vi "AutoRoutinePreProcessor.vi"(1 "MotionPlanningNotifiers":T1, 2 "RawSteps":T11[](array[typedef])) -> (0 "PreProcessedSteps":T2[](array[typedef]) {"ArmPath"."ExtendTrajectory"."Time (ms)" items=["TrajectoryDuration_0ms"=0, "TrajectoryDuration_5ms"=5, "TrajectoryDuration_10ms"=10, "TrajectoryDuration_20ms"=20, "TrajectoryDuration_30ms"=30, "TrajectoryDuration_40ms"=40, "TrajectoryDuration_50ms"=50, "TrajectoryDuration_100ms"=100]; "ArmPath"."RotateTrajectory"."Time (ms)" items=["TrajectoryDuration_0ms"=0, "TrajectoryDuration_5ms"=5, "TrajectoryDuration_10ms"=10, "TrajectoryDuration_20ms"=20, "TrajectoryDuration_30ms"=30, "TrajectoryDuration_40ms"=40, "TrajectoryDuration_50ms"=50, "TrajectoryDuration_100ms"=100]})   [LabVIEW 2017]
uses:
  TypeDef/AutoStep.ctl
  TypeDef/AutoWaypointType.ctl
  Pathfinder/Pathfinder-LabVIEW/Pathfinder-Lib/VIs/Waypoint.ctl
  Implements/Arm/TypeDefs/ArmTargetPosition.ctl
  Implements/TypeDefs/IntakeState.ctl
  TypeDef/AutoPreProcessedStep.ctl
  PathPlannerSupport/TypeDefs/DrivePlanResponse.ctl
  Pathfinder/Pathfinder-LabVIEW/Pathfinder-Lib/VIs/Segment.ctl
  Implements/Arm/TypeDefs/ArmPlanResponse.ctl
  General/MotionProfiling/TypeDefs/TrajectoryPoint.ctl
  <vilib>/Rock Robotics/WPI/ThirdParty/Phoenix-LabVIEW/Motor Controller/Controls/CTRE_Phoenix_MotorControl_TrajectoryPointTimeDur.ctl
  TypeDefs/RobotComponents/MotionPlanningNotifiers.ctl
  PathPlannerSupport/TypeDefs/DrivePlanRequest.ctl
  Implements/Arm/TypeDefs/ArmPlanRequest.ctl
  Pathfinder/Pathfinder-LabVIEW/Pathfinder-Lib/Pathfinder.lvlib
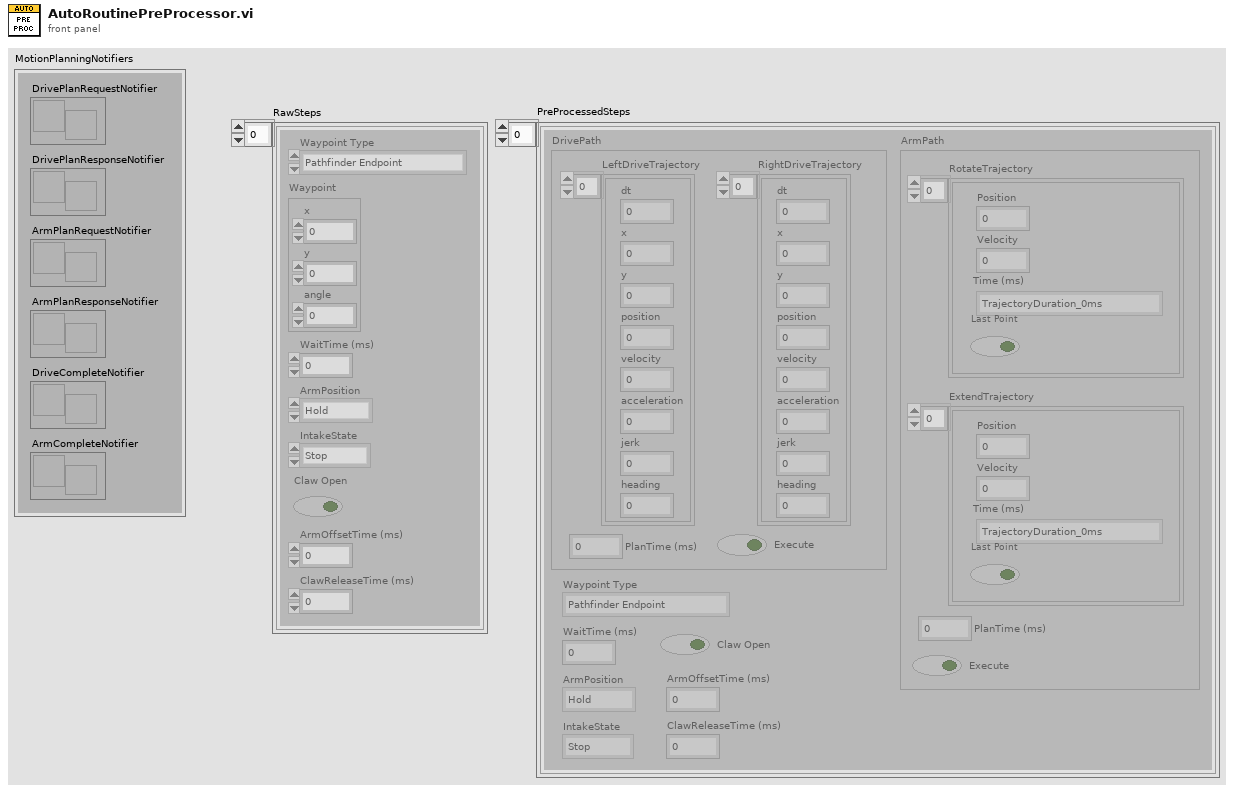
[diagram p1: front panel]
types:
  T1 = typedef "MotionPlanningNotifiers.ctl" = cluster{"DrivePlanRequestNotifier":refnum<notifier>, "DrivePlanResponseNotifier":refnum<notifier>, "ArmPlanRequestNotifier":refnum<notifier>, "ArmPlanResponseNotifier":refnum<notifier>, "DriveCompleteNotifier":refnum<notifier>, "ArmCompleteNotifier":refnum<notifier>}
  T2 = typedef "AutoPreProcessedStep.ctl" = cluster{"DrivePath":T3, "ArmPath":T5, "Waypoint Type":T8, "WaitTime (ms)":u16, "ArmPosition":T9, "IntakeState":T10, "Claw Open":bool, "ArmOffsetTime (ms)":u16, "ClawReleaseTime (ms)":i32}
  T3 = typedef "DrivePlanResponse.ctl" = cluster{"LeftDriveTrajectory":T4[], "RightDriveTrajectory":T4[], "PlanTime (ms)":u32, "Execute":bool}
  T4 = typedef "Pathfinder.lvlib/Segment.ctl" = cluster{"dt":dbl, "x":dbl, "y":dbl, "position":dbl, "velocity":dbl, "acceleration":dbl, "jerk":dbl, "heading":dbl}
  T5 = typedef "ArmPlanResponse.ctl" = cluster{"RotateTrajectory":T6[], "ExtendTrajectory":T6[], "PlanTime (ms)":u32, "Execute":bool}
  T6 = typedef "TrajectoryPoint.ctl" = cluster{"Position ":dbl, "Velocity ":dbl, "Time (ms)":T7, "Last Point":bool}
  T7 = typedef "CTRE_Phoenix_MotorControl_TrajectoryPointTimeDur.ctl" = i32
  T8 = typedef "AutoWaypointType.ctl" = enum16{"Pathfinder Endpoint", "Pathfinder Waypoint", "Zero-Radius Turn Endpoint", "Stationary", "Vision Assist Endpoint", "Stop"}
  T9 = typedef "ArmTargetPosition.ctl" = enum16{"Hold", "Switch", "Scale Low", "Scale High", "Climb", "Back Place"}
  T10 = typedef "IntakeState.ctl" = enum16{"Stop", "Forward", "Reverse", "Forward Open"}
  T11 = typedef "AutoStep.ctl" = cluster{"Waypoint Type":T8, "Waypoint":T12, "WaitTime (ms)":u16, "ArmPosition":T9, "IntakeState":T10, "Claw Open":bool, "ArmOffsetTime (ms)":u16, "ClawReleaseTime (ms)":i32}
  T12 = typedef "Pathfinder.lvlib/Waypoint.ctl" = cluster{"x":dbl, "y":dbl, "angle":dbl}
  T13 = typedef "ArmPlanRequest.ctl" = cluster{"Destination":T9, "Preview":bool, "Start":T9, "Fixed Start":bool}
  T14 = typedef "DrivePlanRequest.ctl" = cluster{"Plan Type":T8, "Waypoints":T12[], "Preview":bool}
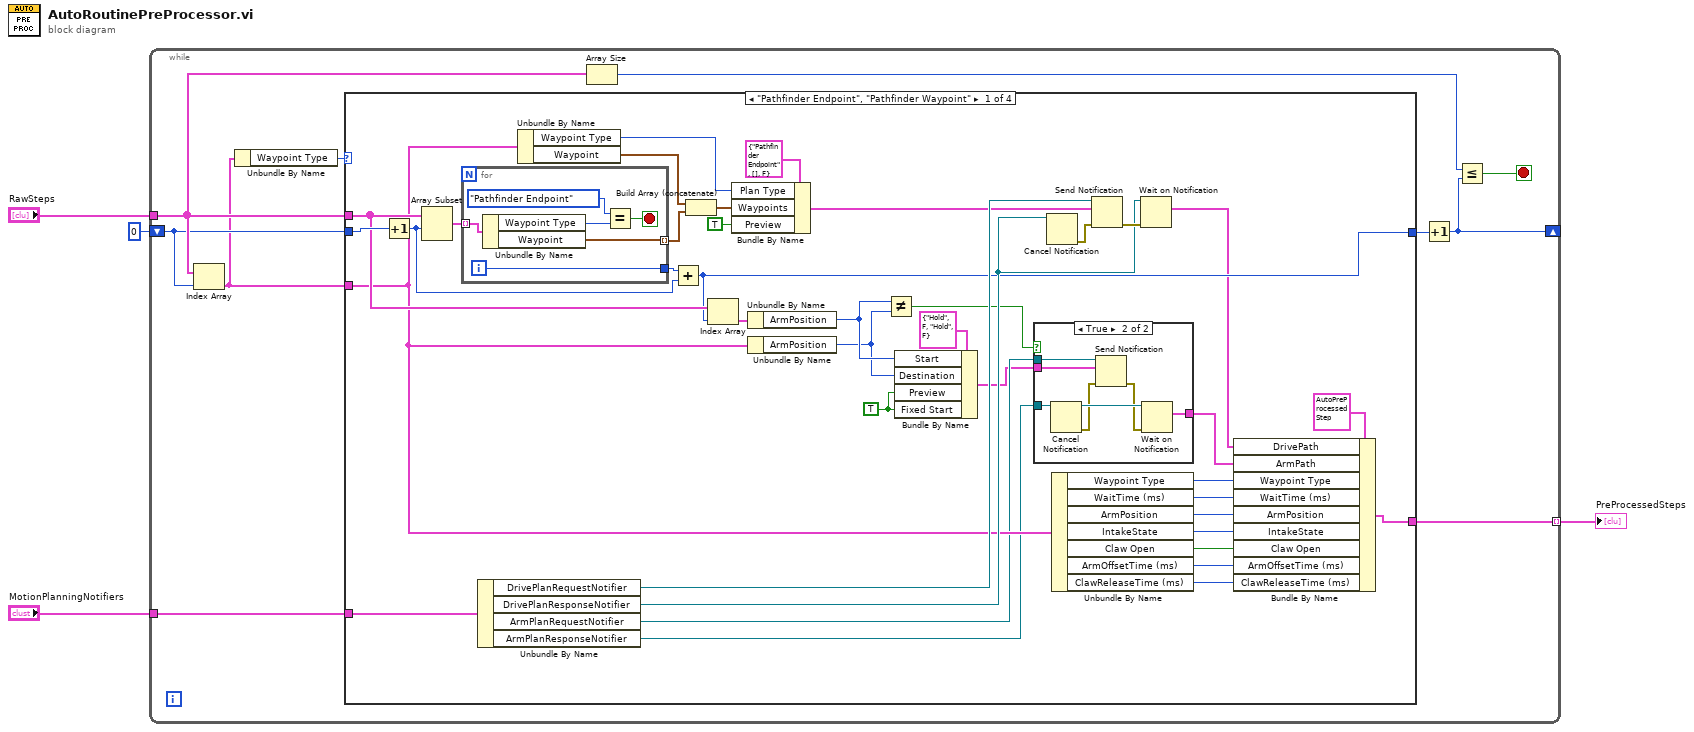
[diagram p0: block diagram]
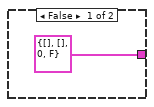
[diagram p2: hidden frame]
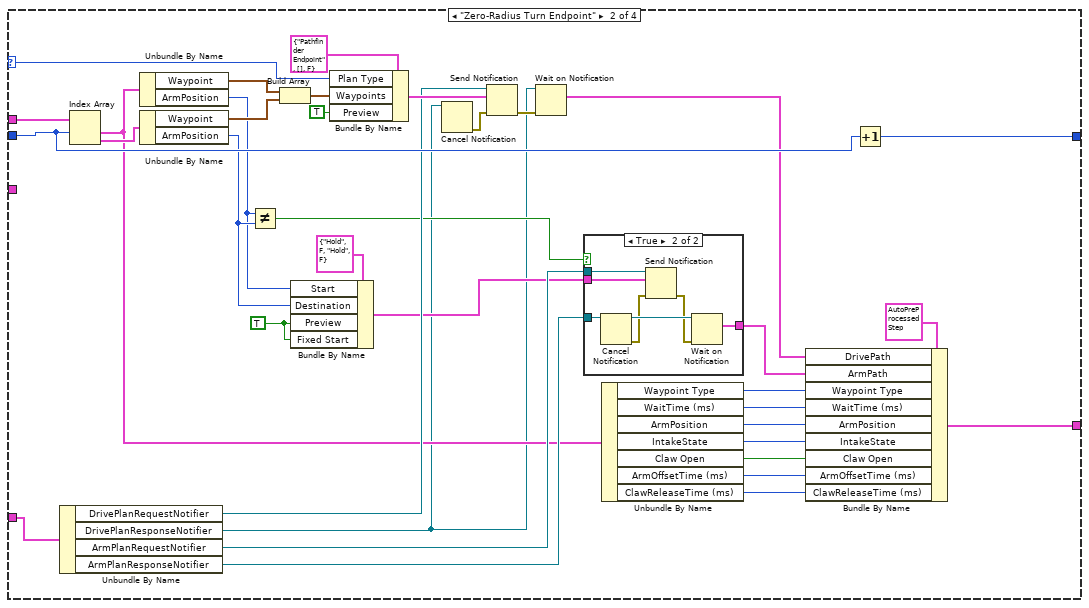
[diagram p3: hidden frame]
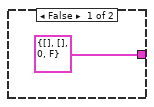
[diagram p4: hidden frame]
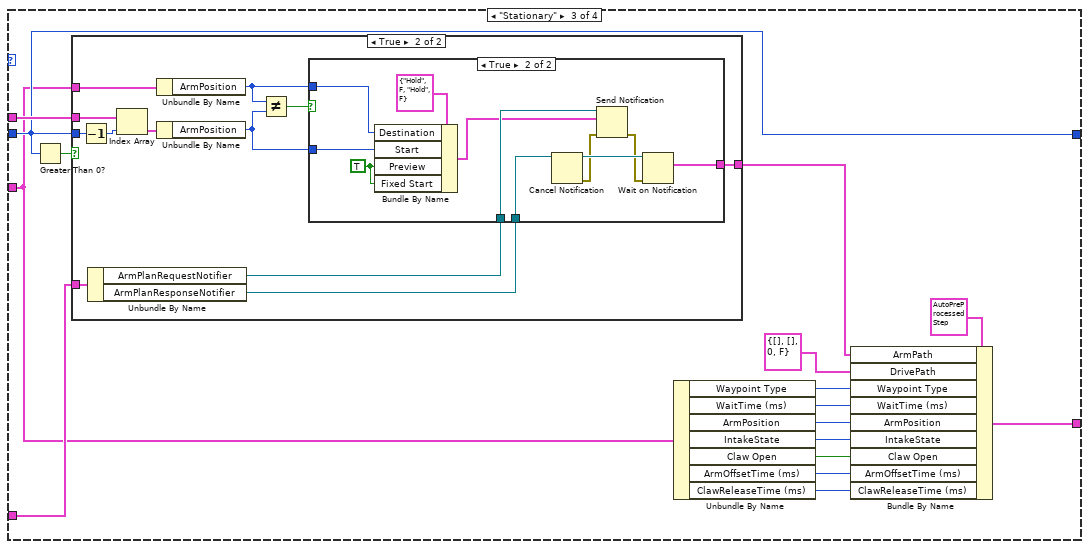
[diagram p5: hidden frame]
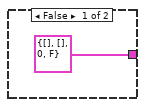
[diagram p6: hidden frame]
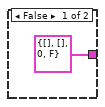
[diagram p7: hidden frame]
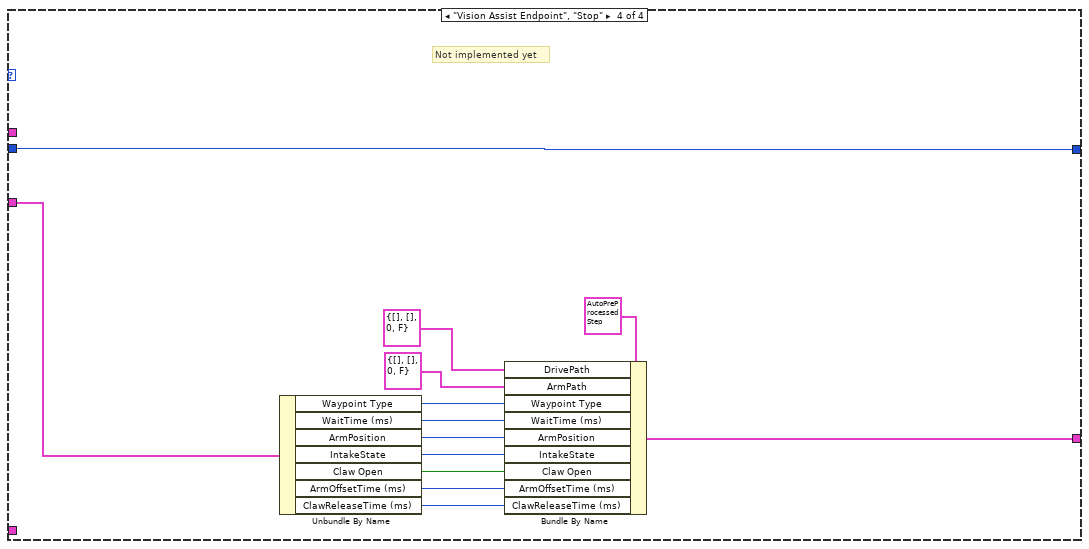
[diagram p8: hidden frame]
diagram:
  n1 = while {
    tunnel: "RawSteps" -> [w9]
    tunnel: "MotionPlanningNotifiers" -> [w14]
    shift-right: [w12] -> _
    shift-left: 0 -> [w8]
    tunnel: [w7] -> w1 mode=indexing
    stop <- w10 stop-if-true
    n2 = Index Array(array=w9, index=w8) -> (element=w6:T11)
    n3 = Unbundle By Name(w6) -> ("Waypoint Type"=w5:T8)
    n4 = case shown="\"Pathfinder Endpoint\", \"Pathfinder Waypoint\"" w5 {
      selector: w5 -> [_ w72 _ _]
      tunnel: w9 -> [w41 w103 w126 _]
      tunnel: w8 -> [w42 w101 w124 w165]
      tunnel: w6 -> [w24 _ w123 w162]
      tunnel: [w18 w102 w124 w165] -> w13
      tunnel: w14 -> [w43 w94 w125 _]
      tunnel: [w19 w71 w121 w163] -> w7
      frame "Pathfinder Endpoint", "Pathfinder Waypoint" {
        w15 = TRUE ("Preview")
        n5 = Increment(x=w42) -> (x+1=w51:i32)
        n6 = Array Subset(array=w41, index=w51) -> (w53:T11[])  [unwired: 1 in]
        n7 = for {
          tunnel: w53 -> [w67] mode=indexing
          tunnel: [w63] -> w52
          tunnel: [w62] -> w47 mode=indexing
          i -> [w63]
          stop <- w64 stop-if-true
          n8 = Unbundle By Name(w67) -> ("Waypoint Type"=w66:T8, "Waypoint"=w62:T12)
          n9 = Equal?(x=AutoWaypointType."Pathfinder Endpoint", y=w66) -> (x = y?=w64:bool)
        }
        n10 = Unbundle By Name(w43) -> ("DrivePlanRequestNotifier"=w36:refnum<notifier>, "DrivePlanResponseNotifier"=w35:refnum<notifier>, "ArmPlanRequestNotifier"=w21:refnum<notifier>, "ArmPlanResponseNotifier"=w22:refnum<notifier>)
        n11 = Unbundle By Name(w24) -> ("Waypoint Type"=w49:T8, "Waypoint"=w48:T12)
        n12 = Add(x=w52, y=w51) -> (x+y=w18:i32)
        n13 = Build Array (concatenate)(w48, w47) -> (w46:T12[])
        n14 = Index Array(array=w41, index=w18) -> (element=w40:T11)
        n15 = Bundle By Name(cluster=T14 {"Plan Type"=enum."Pathfinder Endpoint", "Waypoints"=[], "Preview"=FALSE} ("DrivePlanRequest"), "Plan Type"=w49, "Waypoints"=w46, "Preview"=TRUE) -> (w34:T14)
        n16 = Unbundle By Name(w40) -> ("ArmPosition"=w39:T9)
        n17 = Unbundle By Name(w24) -> ("ArmPosition"=w16:T9)
        n18 = Not Equal?(x=w39, y=w16) -> (x != y?=w23:bool)
        n19 = Bundle By Name(cluster=T13 {"Destination"=enum."Hold", "Preview"=FALSE, "Start"=enum."Hold", "Fixed Start"=FALSE} ("ArmPlanRequest"), "Start"=w39, "Destination"=w16, "Preview"=w15, "Fixed Start"=w15) -> (w20:T13)
        n20 = case shown="True" w23 {
          tunnel: w21 -> [_ w61]
          tunnel: w20 -> [_ w60]
          tunnel: w22 -> [_ w59]
          tunnel: [T5 {"RotateTrajectory"=[], "ExtendTrajectory"=[], "PlanTime (ms)"=0, "Execute"=FALSE} ("ArmPlanResponse") w55] -> w26
          frame False {
          }
          frame True {
            n21 = Cancel Notification(0:w59) -> (8:w58:refnum<notifier>, 11:w57:errorcluster)  [unwired: 1 in, 1 out]
            n22 = Send Notification(notification=w60, notifier=w61, error in (no error)=w57) -> (error out=w56:errorcluster)  [unwired: 1 out]
            n23 = Wait on Notification(notifier=w58, error in (no error)=w56) -> (notification=w55:T5)  [unwired: 2 in, 3 out]
          }
        }
        n24 = Cancel Notification(0:w35) -> (11:w37:errorcluster)  [unwired: 1 in, 2 out]
        n25 = Unbundle By Name(w24) -> ("Waypoint Type"=w25:T8, "WaitTime (ms)"=w27:u16, "ArmPosition"=w28:T9, "IntakeState"=w29:T10, "Claw Open"=w30:bool, "ArmOffsetTime (ms)"=w31:u16, "ClawReleaseTime (ms)"=w32:i32)
        n26 = Send Notification(notification=w34, notifier=w36, error in (no error)=w37) -> (error out=w38:errorcluster)  [unwired: 1 out]
        n27 = Wait on Notification(notifier=w35, error in (no error)=w38) -> (notification=w17:T3)  [unwired: 2 in, 3 out]
        n28 = Bundle By Name(cluster=T2 {"DrivePath"={"LeftDriveTrajectory"=[], "RightDriveTrajectory"=[], "PlanTime (ms)"=0, "Execute"=FALSE}, "ArmPath"={"RotateTrajectory"=[], "ExtendTrajectory"=[], "PlanTime (ms)"=0, "Execute"=FALSE}, "Waypoint Type"=enum."Pathfinder Endpoint", "WaitTime (ms)"=0, "ArmPosition"=enum."Hold", "IntakeState"=enum."Stop", "Claw Open"=FALSE, "ArmOffsetTime (ms)"=0, "ClawReleaseTime (ms)"=0} ("Cluster"), "DrivePath"=w17, "ArmPath"=w26, "Waypoint Type"=w25, "WaitTime (ms)"=w27, "ArmPosition"=w28, "IntakeState"=w29, "Claw Open"=w30, "ArmOffsetTime (ms)"=w31, "ClawReleaseTime (ms)"=w32) -> (w19:T2)
      }
      frame "Zero-Radius Turn Endpoint" {
        w80 = TRUE ("Preview")
        n29 = Unbundle By Name(w94) -> ("DrivePlanRequestNotifier"=w93:refnum<notifier>, "DrivePlanResponseNotifier"=w82:refnum<notifier>, "ArmPlanRequestNotifier"=w91:refnum<notifier>, "ArmPlanResponseNotifier"=w87:refnum<notifier>)
        n30 = Index Array(array=w103, index #1=w101) -> (element #1=w85:T11, element #2=w86:T11)  [unwired: 1 in]
        n31 = Unbundle By Name(w85) -> ("Waypoint"=w99:T12, "ArmPosition"=w81:T9)
        n32 = Unbundle By Name(w86) -> ("Waypoint"=w98:T12, "ArmPosition"=w89:T9)
        n33 = Not Equal?(x=w81, y=w89) -> (x != y?=w88:bool)
        n34 = Build Array(w99, w98) -> (w97:T12[])
        n35 = Bundle By Name(cluster=T13 {"Destination"=enum."Hold", "Preview"=FALSE, "Start"=enum."Hold", "Fixed Start"=FALSE} ("ArmPlanRequest"), "Start"=w81, "Destination"=w89, "Preview"=w80, "Fixed Start"=w80) -> (w90:T13)
        n36 = Bundle By Name(cluster=T14 {"Plan Type"=enum."Pathfinder Endpoint", "Waypoints"=[], "Preview"=FALSE} ("DrivePlanRequest"), "Plan Type"=w72, "Waypoints"=w97, "Preview"=TRUE) -> (w96:T14)
        n37 = Cancel Notification(0:w82) -> (11:w83:errorcluster)  [unwired: 1 in, 2 out]
        n38 = Send Notification(notification=w96, notifier=w93, error in (no error)=w83) -> (error out=w84:errorcluster)  [unwired: 1 out]
        n39 = Wait on Notification(notifier=w82, error in (no error)=w84) -> (notification=w70:T3)  [unwired: 2 in, 3 out]
        n40 = case shown="True" w88 {
          tunnel: w91 -> [_ w111]
          tunnel: w90 -> [_ w110]
          tunnel: w87 -> [_ w109]
          tunnel: [T5 {"RotateTrajectory"=[], "ExtendTrajectory"=[], "PlanTime (ms)"=0, "Execute"=FALSE} ("ArmPlanResponse") w105] -> w69
          frame False {
          }
          frame True {
            n41 = Cancel Notification(0:w109) -> (8:w108:refnum<notifier>, 11:w107:errorcluster)  [unwired: 1 in, 1 out]
            n42 = Send Notification(notification=w110, notifier=w111, error in (no error)=w107) -> (error out=w106:errorcluster)  [unwired: 1 out]
            n43 = Wait on Notification(notifier=w108, error in (no error)=w106) -> (notification=w105:T5)  [unwired: 2 in, 3 out]
          }
        }
        n44 = Unbundle By Name(w85) -> ("Waypoint Type"=w68:T8, "WaitTime (ms)"=w73:u16, "ArmPosition"=w74:T9, "IntakeState"=w75:T10, "Claw Open"=w76:bool, "ArmOffsetTime (ms)"=w77:u16, "ClawReleaseTime (ms)"=w78:i32)
        n45 = Bundle By Name(cluster=T2 {"DrivePath"={"LeftDriveTrajectory"=[], "RightDriveTrajectory"=[], "PlanTime (ms)"=0, "Execute"=FALSE}, "ArmPath"={"RotateTrajectory"=[], "ExtendTrajectory"=[], "PlanTime (ms)"=0, "Execute"=FALSE}, "Waypoint Type"=enum."Pathfinder Endpoint", "WaitTime (ms)"=0, "ArmPosition"=enum."Hold", "IntakeState"=enum."Stop", "Claw Open"=FALSE, "ArmOffsetTime (ms)"=0, "ClawReleaseTime (ms)"=0} ("Cluster"), "DrivePath"=w70, "ArmPath"=w69, "Waypoint Type"=w68, "WaitTime (ms)"=w73, "ArmPosition"=w74, "IntakeState"=w75, "Claw Open"=w76, "ArmOffsetTime (ms)"=w77, "ClawReleaseTime (ms)"=w78) -> (w71:T2)
        n46 = Increment(x=w101) -> (x+1=w102:i32)
      }
      frame "Stationary" {
        n47 = Greater Than 0?(x=w124) -> (x > 0?=w127:bool)
        n48 = case shown="True" w127 {
          tunnel: w126 -> [_ w140]
          tunnel: w124 -> [_ w139]
          tunnel: w123 -> [_ w136]
          tunnel: w125 -> [_ w134]
          tunnel: [T5 {"RotateTrajectory"=[], "ExtendTrajectory"=[], "PlanTime (ms)"=0, "Execute"=FALSE} ("ArmPlanResponse") w129] -> w113
          frame False {
          }
          frame True {
            n49 = Decrement(x=w139) -> (x-1=w138:i32)
            n50 = Unbundle By Name(w134) -> ("ArmPlanRequestNotifier"=w133:refnum<notifier>, "ArmPlanResponseNotifier"=w131:refnum<notifier>)
            n51 = Index Array(array=w140, index=w138) -> (element=w137:T11)
            n52 = Unbundle By Name(w136) -> ("ArmPosition"=w132:T9)
            n53 = Unbundle By Name(w137) -> ("ArmPosition"=w130:T9)
            n54 = Not Equal?(x=w132, y=w130) -> (x != y?=w135:bool)
            n55 = case shown="True" w135 {
              tunnel: w133 -> [_ w148]
              tunnel: w132 -> [_ w145]
              tunnel: w131 -> [_ w147]
              tunnel: w130 -> [_ w144]
              tunnel: [T5 {"RotateTrajectory"=[], "ExtendTrajectory"=[], "PlanTime (ms)"=0, "Execute"=FALSE} ("ArmPlanResponse") w142] -> w129
              frame False {
              }
              frame True {
                w143 = TRUE ("Preview")
                n56 = Bundle By Name(cluster=T13 {"Destination"=enum."Hold", "Preview"=FALSE, "Start"=enum."Hold", "Fixed Start"=FALSE} ("notification"), "Destination"=w145, "Start"=w144, "Preview"=w143, "Fixed Start"=w143) -> (w146:T13)
                n57 = Cancel Notification(0:w147) -> (8:w151:refnum<notifier>, 11:w150:errorcluster)  [unwired: 1 in, 1 out]
                n58 = Send Notification(notification=w146, notifier=w148, error in (no error)=w150) -> (error out=w149:errorcluster)  [unwired: 1 out]
                n59 = Wait on Notification(notifier=w151, error in (no error)=w149) -> (notification=w142:T5)  [unwired: 2 in, 3 out]
              }
            }
          }
        }
        n60 = Unbundle By Name(w123) -> ("Waypoint Type"=w112:T8, "WaitTime (ms)"=w115:u16, "ArmPosition"=w116:T9, "IntakeState"=w117:T10, "Claw Open"=w118:bool, "ArmOffsetTime (ms)"=w119:u16, "ClawReleaseTime (ms)"=w120:i32)
        n61 = Bundle By Name(cluster=T2 {"DrivePath"={"LeftDriveTrajectory"=[], "RightDriveTrajectory"=[], "PlanTime (ms)"=0, "Execute"=FALSE}, "ArmPath"={"RotateTrajectory"=[], "ExtendTrajectory"=[], "PlanTime (ms)"=0, "Execute"=FALSE}, "Waypoint Type"=enum."Pathfinder Endpoint", "WaitTime (ms)"=0, "ArmPosition"=enum."Hold", "IntakeState"=enum."Stop", "Claw Open"=FALSE, "ArmOffsetTime (ms)"=0, "ClawReleaseTime (ms)"=0} ("Cluster"), "ArmPath"=w113, "DrivePath"=T3 {"LeftDriveTrajectory"=[], "RightDriveTrajectory"=[], "PlanTime (ms)"=0, "Execute"=FALSE}, "Waypoint Type"=w112, "WaitTime (ms)"=w115, "ArmPosition"=w116, "IntakeState"=w117, "Claw Open"=w118, "ArmOffsetTime (ms)"=w119, "ClawReleaseTime (ms)"=w120) -> (w121:T2)
      }
      frame "Vision Assist Endpoint", "Stop" {
        # "Not implemented yet"
        n62 = Unbundle By Name(w162) -> ("Waypoint Type"=w155:T8, "WaitTime (ms)"=w156:u16, "ArmPosition"=w157:T9, "IntakeState"=w158:T10, "Claw Open"=w159:bool, "ArmOffsetTime (ms)"=w160:u16, "ClawReleaseTime (ms)"=w161:i32)
        n63 = Bundle By Name(cluster=T2 {"DrivePath"={"LeftDriveTrajectory"=[], "RightDriveTrajectory"=[], "PlanTime (ms)"=0, "Execute"=FALSE}, "ArmPath"={"RotateTrajectory"=[], "ExtendTrajectory"=[], "PlanTime (ms)"=0, "Execute"=FALSE}, "Waypoint Type"=enum."Pathfinder Endpoint", "WaitTime (ms)"=0, "ArmPosition"=enum."Hold", "IntakeState"=enum."Stop", "Claw Open"=FALSE, "ArmOffsetTime (ms)"=0, "ClawReleaseTime (ms)"=0} ("Cluster"), "DrivePath"=T3 {"LeftDriveTrajectory"=[], "RightDriveTrajectory"=[], "PlanTime (ms)"=0, "Execute"=FALSE}, "ArmPath"=T5 {"RotateTrajectory"=[], "ExtendTrajectory"=[], "PlanTime (ms)"=0, "Execute"=FALSE}, "Waypoint Type"=w155, "WaitTime (ms)"=w156, "ArmPosition"=w157, "IntakeState"=w158, "Claw Open"=w159, "ArmOffsetTime (ms)"=w160, "ClawReleaseTime (ms)"=w161) -> (w163:T2)
      }
    }
    n64 = Array Size(array=w9) -> (size(s)=w11:i32)
    n65 = Increment(x=w13) -> (x+1=w12:i32)
    n66 = Less Or Equal?(x=w11, y=w12) -> (x <= y?=w10:bool)
  }
  "PreProcessedSteps" <- w1
